vi "m1m3_logEvent_PowerStatus.vi"(8 "error in (no error)":errorcluster, 11 "logevent_PowerStatus_Ctl":T1) -> (0 "error out":errorcluster, 2 "function return":i32, 3 "logevent_PowerStatus_Ctl out":T1)   [LabVIEW 2016, in "SALLV_m1m3.lvlib"]
doc: "int m1m3_shm_logEvent_PowerStatusLV(m1m3_logevent_PowerStatusLV *logevent_PowerStatus_Ctl );"
uses:
  SALLV_m1m3.lvlib
  DataTypes/logevent_PowerStatus.ctl
  SALLV_m1m3.so
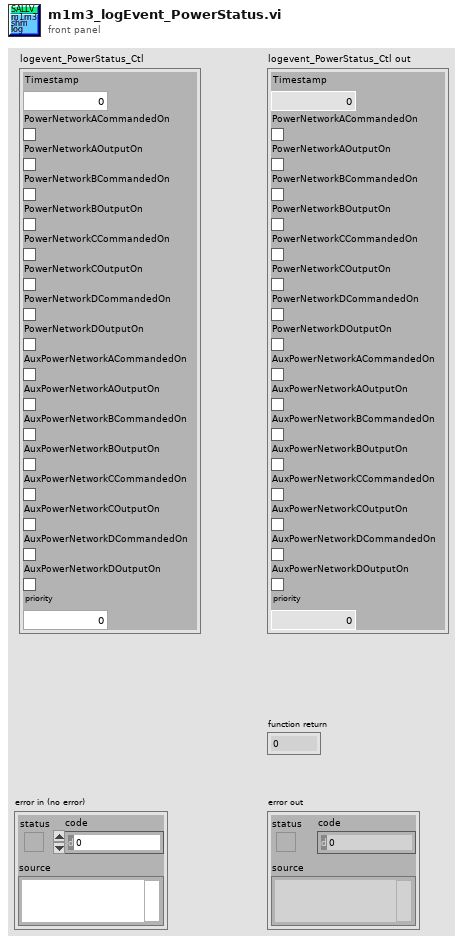
[diagram p1: front panel]
types:
  T1 = typedef "SALLV_m1m3.lvlib/logevent_PowerStatus.ctl" = cluster{"Timestamp":dbl, "PowerNetworkACommandedOn":bool, "PowerNetworkAOutputOn":bool, "PowerNetworkBCommandedOn":bool, "PowerNetworkBOutputOn":bool, "PowerNetworkCCommandedOn":bool, "PowerNetworkCOutputOn":bool, "PowerNetworkDCommandedOn":bool, "PowerNetworkDOutputOn":bool, "AuxPowerNetworkACommandedOn":bool, "AuxPowerNetworkAOutputOn":bool, "AuxPowerNetworkBCommandedOn":bool, "AuxPowerNetworkBOutputOn":bool, "AuxPowerNetworkCCommandedOn":bool, "AuxPowerNetworkCOutputOn":bool, "AuxPowerNetworkDCommandedOn":bool, "AuxPowerNetworkDOutputOn":bool, "priority":i32}
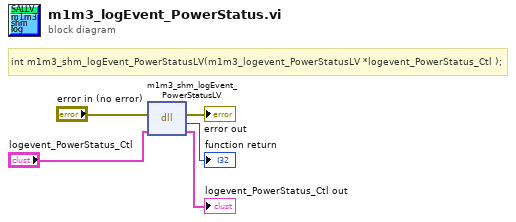
[diagram p0: block diagram]
diagram:
  # "int m1m3_shm_logEvent_PowerStatusLV(m1m3_logevent_PowerStatusLV *logevent_PowerStatus_Ctl );"
  n1 = dll-call lib="opt/CODE/SALLV_m1m3/SALLV_m1m3.*" fn="m1m3_shm_logEvent_PowerStatusLV"(error in="error in (no error)", "logevent_PowerStatus_Ctl"="logevent_PowerStatus_Ctl") -> (error out=→"error out":errorcluster, →"function return":i32, "logevent_PowerStatus_Ctl"=→"logevent_PowerStatus_Ctl out":T1)  [unwired: 2 in, 1 out]
